vi "Init UI Refs.vi"(8 "error in (no error)":errorcluster, 11 "UI in":refnum<class "UI.lvclass">) -> (0 "error out":errorcluster, 3 "UI out":refnum<class "UI.lvclass">)   [LabVIEW 2015, in "UI.lvlib" / "UI.lvclass"]
uses:
  UI.lvclass
  UI.lvclass/UI.ctl
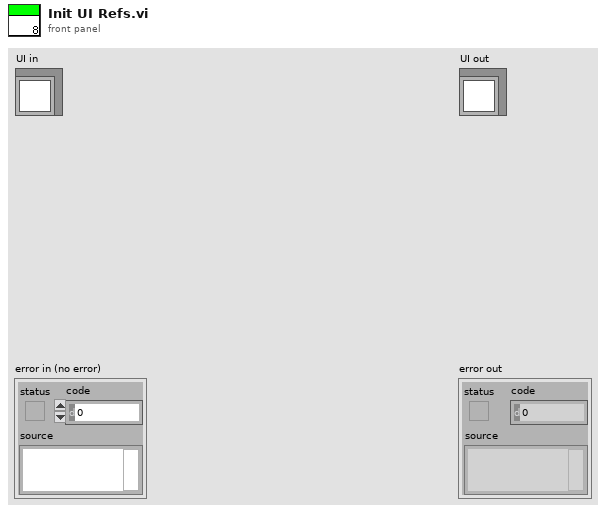
[diagram p1: front panel]
types:
  T1 = enum8{"Enabled", "Disabled", "Disabled and Grayed Out"}
  T2 = typedef "UI.lvlib/UI.lvclass/Ctl Refs.ctl" = cluster{"Basic Params":refnum<vi>, "Type":refnum<vi>, "Channel":refnum<vi>, "Device":refnum<vi>, "Used Channels":refnum<vi>, "Add Channel":refnum<vi>, "Stop Program":refnum<vi>, "Delete Channels":refnum<vi>}
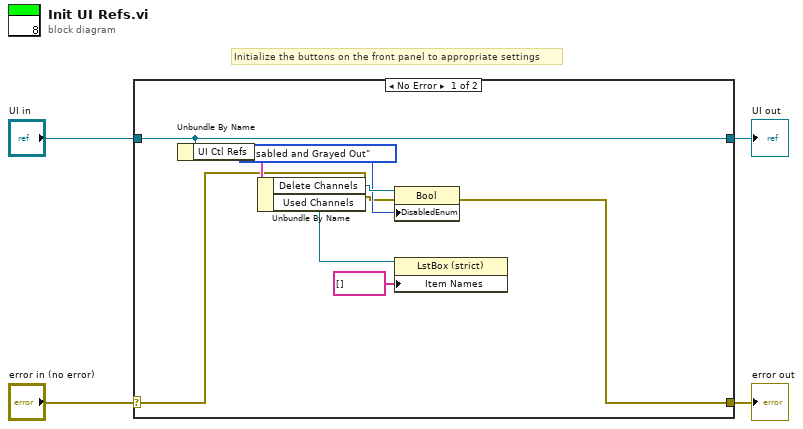
[diagram p0: block diagram]
diagram:
  # "Initialize the buttons on the front panel to appropriate settings"
  n1 = case shown="No Error" "error in (no error)" {
    selector: "error in (no error)" -> [w8 w14]
    tunnel: [w7 w14] -> w3
    tunnel: [w12 w13] -> w1
    tunnel: "UI in" -> [w12 w13]
    frame No Error {
      n2 = Unbundle By Name(w12) -> ("UI Ctl Refs"=w11:T2)
      n3 = Unbundle By Name(w11) -> ("Delete Channels"=w10:refnum<vi>, "Used Channels"=w6:refnum<vi>)
      n4 = property class="Bool"(reference=w10, error in=w8, "DisabledEnum"=T1."Disabled and Grayed Out" ("Disabled")) -> (error out=w7:errorcluster)  [unwired: 1 out]
      n5 = property class="LstBox (strict)"(reference=w6, "Item Names"=string[] []) -> ()  [unwired: 1 in, 2 out]
    }
    frame Error {
    }
  }
  "error out" <- w3
  "UI out" <- w1
